vi "INFO.vi"(0 "TCP session out":refnum<k5>, 2 "Option":T1(ring), 11 "error in":errorcluster) -> (4 "TCP session out":refnum<k5>, 6 "Data":T2, 15 "error out":errorcluster)   [LabVIEW 2023]
uses:
  SubVIs/Controls/redis-data.ctl
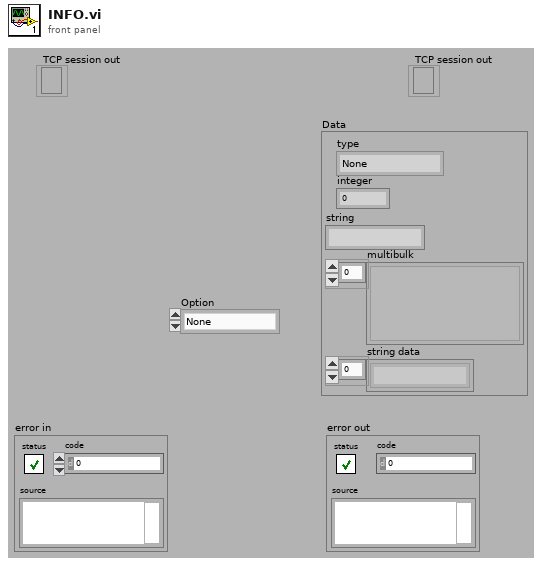
[diagram p1: front panel]
types:
  T1 = enum16{"None", "SERVER", "CLIENTS", "MEMORY", "PERSISTENCE", "STATS", "REPLICATION", "CPU", "COMMANDSTATS", "CLUSTER", "KEYSPACE", "ALL", "DEFAULT"}
  T2 = typedef "redis-data.ctl" = cluster{"type":enum16{"None", "Error", "Status", "Nil", "Integer", "String", "Multibulk"}, "integer":i64, "string":string, "multibulk":variant[], "string data":string[]}
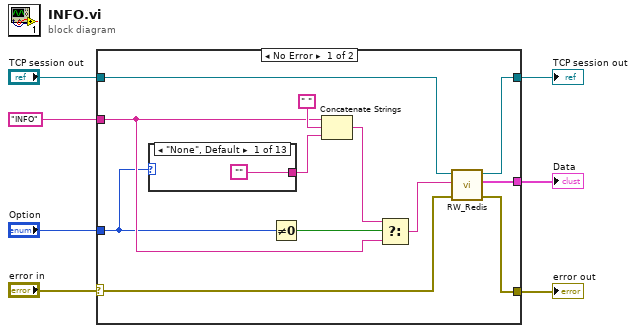
[diagram p0: block diagram]
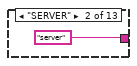
[diagram p2: hidden frame]
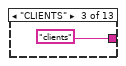
[diagram p3: hidden frame]
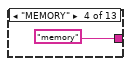
[diagram p4: hidden frame]
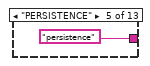
[diagram p5: hidden frame]
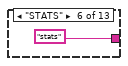
[diagram p6: hidden frame]
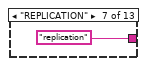
[diagram p7: hidden frame]
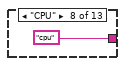
[diagram p8: hidden frame]
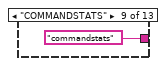
[diagram p9: hidden frame]
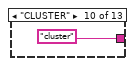
[diagram p10: hidden frame]
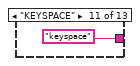
[diagram p11: hidden frame]
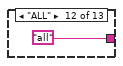
[diagram p12: hidden frame]
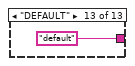
[diagram p13: hidden frame]
diagram:
  n1 = case shown="No Error" "error in" {
    selector: "error in" -> [w19 w34]
    tunnel: "INFO" -> [w10 _]
    tunnel: "TCP session out" -> [w16 w33]
    tunnel: [w18 w34] -> w5
    tunnel: [w17 _] -> w2
    tunnel: [w8 w33] -> w4
    tunnel: "Option" -> [w9 _]
    frame No Error {
      n2 = case shown="\"None\", Default" w9 {
        tunnel: ["" "server" "clients" "memory" "persistence" "stats" "replication" "cpu" "commandstats" "cluster" "keyspace" "all" "default"] -> w13
        frame "None", Default {
        }
        frame "SERVER" {
        }
        frame "CLIENTS" {
        }
        frame "MEMORY" {
        }
        frame "PERSISTENCE" {
        }
        frame "STATS" {
        }
        frame "REPLICATION" {
        }
        frame "CPU" {
        }
        frame "COMMANDSTATS" {
        }
        frame "CLUSTER" {
        }
        frame "KEYSPACE" {
        }
        frame "ALL" {
        }
        frame "DEFAULT" {
        }
      }
      n3 = Not Equal To 0?(x=w9) -> (x != 0?=w15:bool)
      n4 = Concatenate Strings(w10, " ", w13) -> (w12:string)
      n5 = Select(t=w12, s=w15, f=w10) -> (s? t:f=w11:string)
      n6 = call "RW_Redis.vi"("error in"=w19, "command"=w11, "TCP session in"=w16) -> ("error out"=w18:errorcluster, "Data"=w17:T2, "TCP session out"=w8:refnum<k5>)  [unwired: 6 in]
    }
    frame Error {
    }
  }
  "error out" <- w5
  "Data" <- w2
  "TCP session out" <- w4
